vi "Sprawdz_aktywne_kanaly_pom.vi"(7 "Kanaly pom":i32[](array[numeric]), 8 "error in (no error)":errorcluster, 10 "Wolna In":T1 {"Rej.8"."Wolna Wykr num" items=["Brak", "Wykres 1", "Wykres 2", "Wykres 3", "Wykres 4"]; "Rej.7"."Wolna Wykr num" items=["Brak", "Wykres 1", "Wykres 2", "Wykres 3", "Wykres 4"]; "Rej.6"."Wolna Wykr num" items=["Brak", "Wykres 1", "Wykres 2", "Wykres 3", "Wykres 4"]; "Rej.5"."Wolna Wykr num" items=["Brak", "Wykres 1", "Wykres 2", "Wykres 3", "Wykres 4"]; "Rej.4"."Wolna Wykr num" items=["Brak", "Wykres 1", "Wykres 2", "Wykres 3", "Wykres 4"]; "Rej.3"."Wolna Wykr num" items=["Brak", "Wykres 1", "Wykres 2", "Wykres 3", "Wykres 4"]; "Rej.2"."Wolna Wykr num" items=["Brak", "Wykres 1", "Wykres 2", "Wykres 3", "Wykres 4"]; "Rej.1"."Wolna Wykr num" items=["Brak", "Wykres 1", "Wykres 2", "Wykres 3", "Wykres 4"]; "Czas max" min=2.0; "Okres" min=0.001}) -> (0 "error out":errorcluster, 2 "Wolna Out":T1 {"Rej.8"."Wolna Wykr num" items=["Brak", "Wykres 1", "Wykres 2", "Wykres 3", "Wykres 4"]; "Rej.7"."Wolna Wykr num" items=["Brak", "Wykres 1", "Wykres 2", "Wykres 3", "Wykres 4"]; "Rej.6"."Wolna Wykr num" items=["Brak", "Wykres 1", "Wykres 2", "Wykres 3", "Wykres 4"]; "Rej.5"."Wolna Wykr num" items=["Brak", "Wykres 1", "Wykres 2", "Wykres 3", "Wykres 4"]; "Rej.4"."Wolna Wykr num" items=["Brak", "Wykres 1", "Wykres 2", "Wykres 3", "Wykres 4"]; "Rej.3"."Wolna Wykr num" items=["Brak", "Wykres 1", "Wykres 2", "Wykres 3", "Wykres 4"]; "Rej.2"."Wolna Wykr num" items=["Brak", "Wykres 1", "Wykres 2", "Wykres 3", "Wykres 4"]; "Rej.1"."Wolna Wykr num" items=["Brak", "Wykres 1", "Wykres 2", "Wykres 3", "Wykres 4"]; "Czas max" min=2.0; "Okres" min=0.001})   [LabVIEW 2014]
doc: "Sprawdza czy wszystkie kanały pomiarowe wybrane w kanałach rejestrujących są aktywne"
uses:
  Kontrolki/GUI/Rejestracja_wolna.ctl
  Kontrolki/GUI/RejWol_konfig.ctl
  Kontrolki/GUI/RejWol_typ.ctl
  Kontrolki/GUI/Wolna_WykrNum.ctl
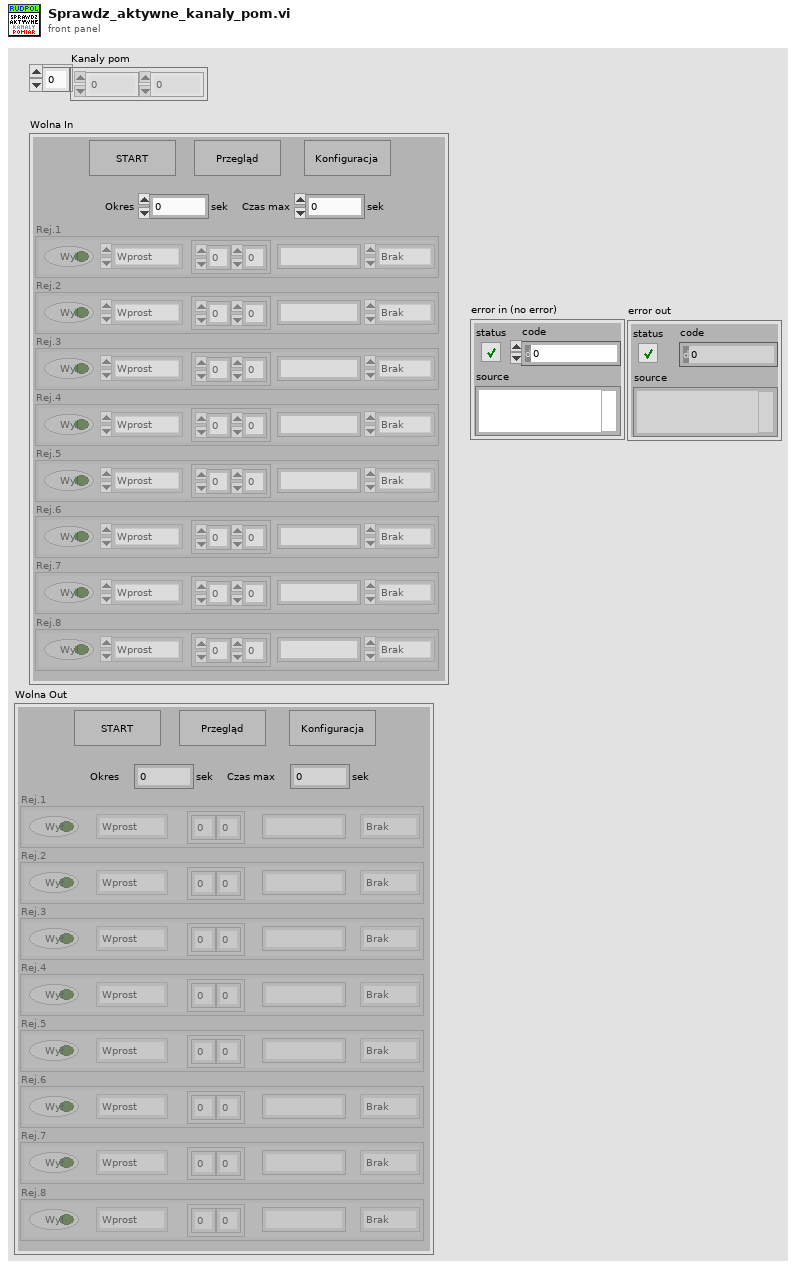
[diagram p1: front panel]
types:
  T1 = typedef "Rejestracja_wolna.ctl" = cluster{"WolnaStart":bool, "WolnaPrzeglad":bool, "Okres":dbl, "Czas max":dbl, "WolnaKonfiguracja":bool, "Rej.1":T2, "Rej.2":T2, "Rej.3":T2, "Rej.4":T2, "Rej.5":T2, "Rej.6":T2, "Rej.7":T2, "Rej.8":T2}
  T2 = typedef "RejWol_konfig.ctl" = cluster{"Typ rejestracji":T3, "Kanały":i32[], "Opis":string, "Aktywny":bool, "Wolna Wykr num":T4}
  T3 = typedef "RejWol_typ.ctl" = enum16{"Wprost", "Moduł", "Kwadrat", "Iloczyn", "Faza"}
  T4 = typedef "Wolna_WykrNum.ctl" = u16
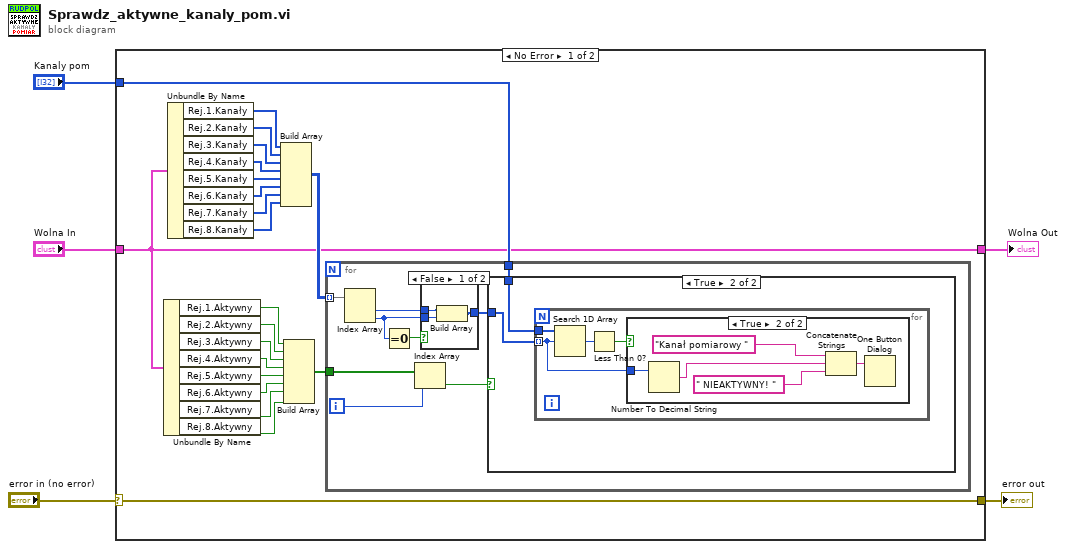
[diagram p0: block diagram]
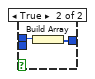
[diagram p2: hidden frame]
diagram:
  n1 = case shown="No Error" "error in (no error)" {
    selector: "error in (no error)" -> [w6 w53]
    tunnel: "Kanaly pom" -> [w26 _]
    tunnel: "Wolna In" -> [w7 w52]
    tunnel: [w7 w52] -> w3
    tunnel: [w6 w53] -> w1
    frame No Error {
      n2 = Unbundle By Name(w7) -> ("Rej.1.Aktywny"=w8:bool, "Rej.2.Aktywny"=w9:bool, "Rej.3.Aktywny"=w10:bool, "Rej.4.Aktywny"=w11:bool, "Rej.5.Aktywny"=w12:bool, "Rej.6.Aktywny"=w13:bool, "Rej.7.Aktywny"=w14:bool, "Rej.8.Aktywny"=w15:bool)
      n3 = Unbundle By Name(w7) -> ("Rej.1.Kanały"=w16:i32[], "Rej.2.Kanały"=w17:i32[], "Rej.3.Kanały"=w18:i32[], "Rej.4.Kanały"=w19:i32[], "Rej.5.Kanały"=w20:i32[], "Rej.6.Kanały"=w21:i32[], "Rej.7.Kanały"=w22:i32[], "Rej.8.Kanały"=w23:i32[])
      n4 = Build Array(w16, w17, w18, w19, w20, w21, w22, w23) -> (w25:i32[][])
      n5 = Build Array(w8, w9, w10, w11, w12, w13, w14, w15) -> (w24:bool[])
      n6 = for {
        tunnel: w24 -> [w35]
        tunnel: w25 -> [w31] mode=indexing
        tunnel: w26 -> [w32]
        i -> [w34]
        n7 = Index Array(array=w31) -> (element #1=w29:i32, element #2=w28:i32)  [unwired: 2 in]
        n8 = Equal To 0?(x=w28) -> (x = 0?=w30:bool)
        n9 = Index Array(array=w35, index=w34) -> (element=w33:bool)
        n10 = case shown="False" w30 {
          tunnel: w29 -> [w38 w39]
          tunnel: w28 -> [w37 _]
          tunnel: [w36 w40] -> w27
          frame False {
            n11 = Build Array(w38, w37) -> (w36:i32[])
          }
          frame True {
            n12 = Build Array(w39) -> (w40:i32[])
          }
        }
        n13 = case shown="True" w33 {
          tunnel: w27 -> [_ w41]
          tunnel: w32 -> [_ w42]
          frame False {
          }
          frame True {
            n14 = for {
              tunnel: w42 -> [w46]
              tunnel: w41 -> [w43] mode=indexing
              n15 = Search 1D Array(1D array=w46, element=w43) -> (index of element=w45:i32)  [unwired: 1 in]
              n16 = Less Than 0?(x=w45) -> (x < 0?=w44:bool)
              n17 = case shown="True" w44 {
                tunnel: w43 -> [_ w48]
                frame False {
                }
                frame True {
                  n18 = Number To Decimal String(number=w48) -> (decimal integer string=w47:string)  [unwired: 1 in]
                  n19 = Concatenate Strings("Kanał pomiarowy " ("message"), w47, " NIEAKTYWNY! " ("message")) -> (w50:string)
                  n20 = One Button Dialog(message=w50) -> ()  [unwired: 1 in, 1 out]
                }
              }
            }
          }
        }
      }
    }
    frame Error {
    }
  }
  "Wolna Out" <- w3
  "error out" <- w1
